vi "bresenham_algorithm.vi"(0 "pX":dbl, 5 "pY":dbl, 7 "speed (ms)":u32(knob) scale=0.0..20.0, 9 "newX":dbl, 11 "newY":dbl) -> ()   [LabVIEW 2016]
panel:
  out "error (dy > dx)":dbl
  out "error (dx >= dy)":dbl
  out "dX":dbl
  out "dY":dbl
  out "direction X":bool[](array[boolean])
  out "direction Y":bool[](array[boolean])
  # "This program let the user to draw a linear line at feed rate.\nThis program implement the Bresenham's line Algorithm. \nUser must enter feed rate in millisecond (ms).\nThe pX and pY is the start points of the linear line.\nThe newX and newY is the end points of the linear line."
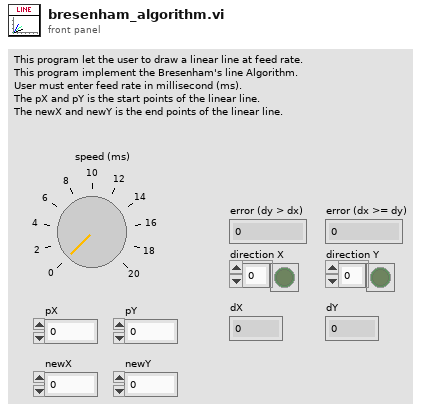
[diagram p1: front panel]
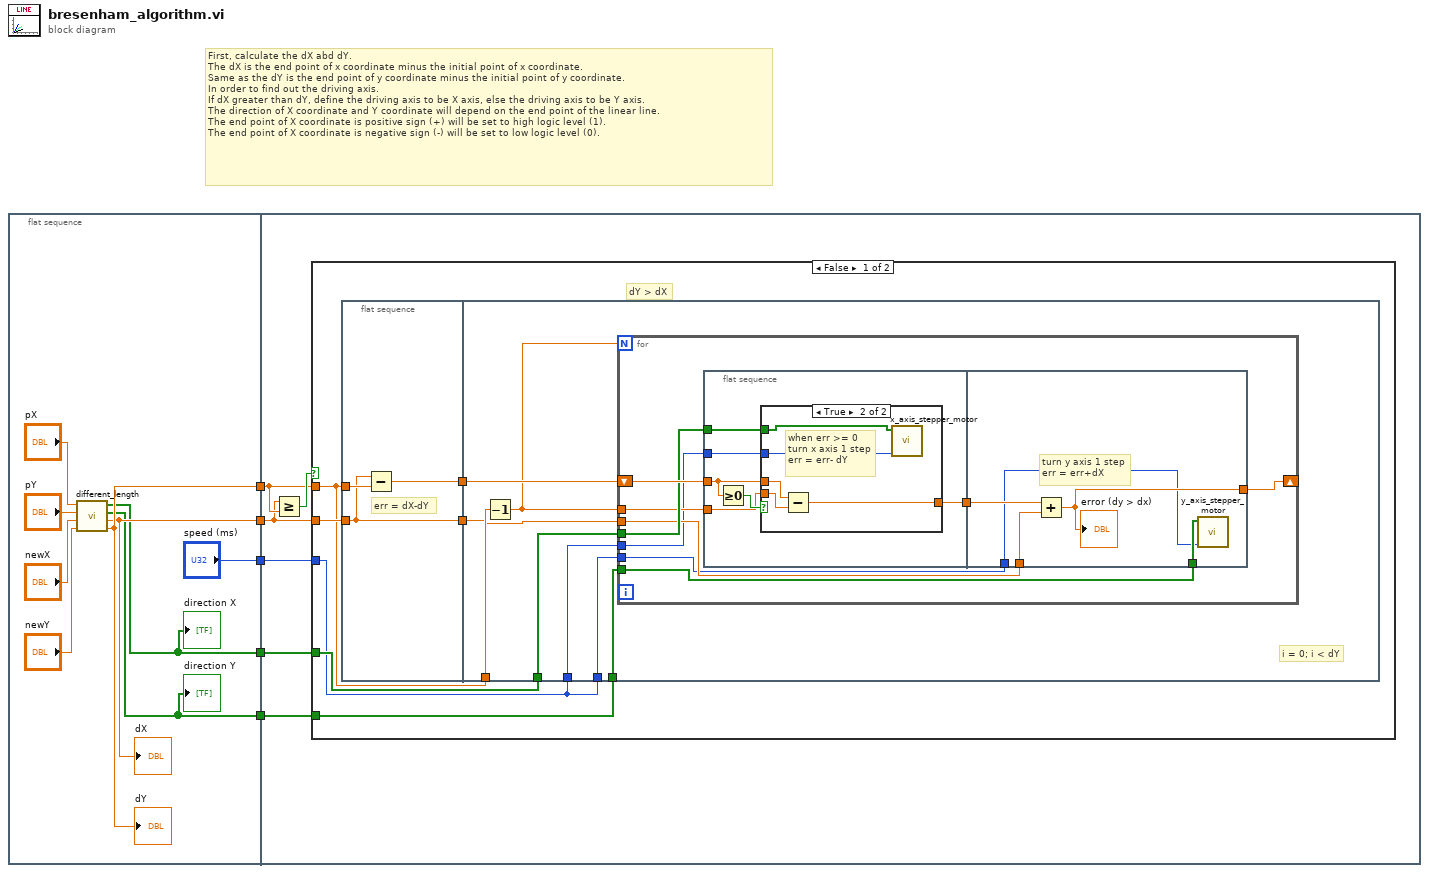
[diagram p0: block diagram]
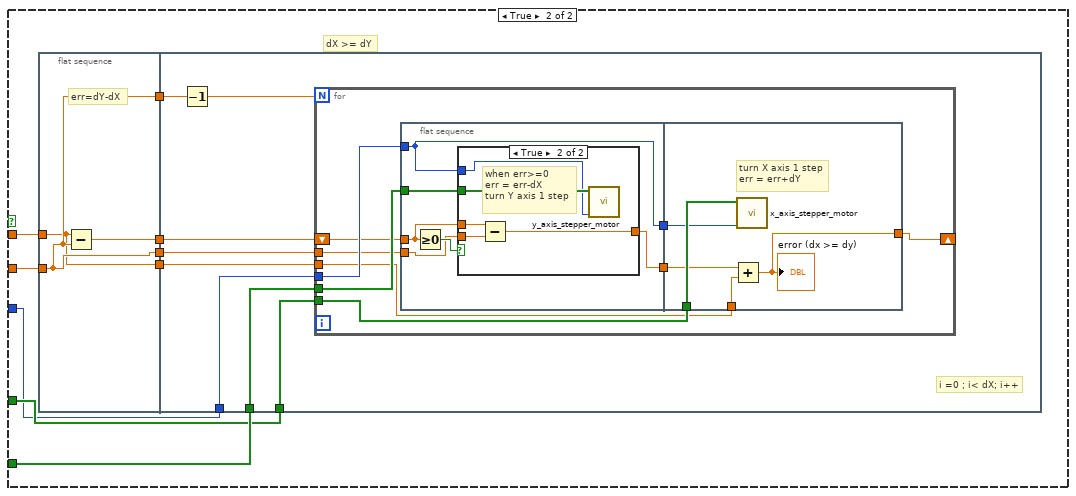
[diagram p3: hidden frame]
diagram:
  # "First, calculate the dX abd dY. \nThe dX is the end point of x coordinate minus the initial point of x coordinate.\nSame as the dY is the end point of y coordinate minus the initial point of y coordinate.\nIn order to find out the driving axis. \nIf dX greater than dY, define the driving axis to be X axis, else the driving axis to be Y axis.\nThe direction of X coordinate and Y coordinate will depend on the end point of the linear line. \nThe end point of X coordinate is positive sign (+) will be set to high logic level (1).\nThe end point of X coordinate is negative sign (-) will be set to low logic level (0)."
  n1 = flat-sequence {
    tunnel: [w12] -> w5
    tunnel: [w11] -> w4
    tunnel: [w10] -> w3
    tunnel: ["speed (ms)"] -> w2
    tunnel: [w13] -> w1
    tunnel: w5 -> [w15]
    tunnel: w4 -> [w19]
    tunnel: w3 -> [w18]
    tunnel: w2 -> [w17]
    tunnel: w1 -> [w16]
    frame #0 {
      n2 = call "different_length.vi"("newY"="newY", "newX"="newX", "pY"="pY", "pX"="pX") -> ("dY"=w13:dbl, "dX"=w12:dbl, "dirY"=w11:bool[], "dirX"=w10:bool[])  [unwired: 4 in]
      "dX" <- w12
      "dY" <- w13
      "direction X" <- w10
      "direction Y" <- w11
    }
    frame #1 {
      n3 = Greater Or Equal?(x=w15, y=w16) -> (x >= y?=w20:bool)
      n4 = case shown="False" w20 {
        tunnel: w19 -> [w26 w73]
        tunnel: w18 -> [w25 w72]
        tunnel: w17 -> [w21 w71]
        tunnel: w16 -> [w23 w69]
        tunnel: w15 -> [w24 w68]
        frame False {
          # "dY > dX"
          n5 = flat-sequence {
            tunnel: [w30] -> w27
            tunnel: w24 -> [w28]
            tunnel: w23 -> [w29]
            tunnel: [w28] -> w22
            tunnel: w27 -> [w38]
            tunnel: w26 -> [w37]
            tunnel: w25 -> [w36]
            tunnel: w23 -> [w35]
            tunnel: w22 -> [w33]
            tunnel: w21 -> [w32]
            tunnel: w21 -> [w31]
            frame #0 {
              # "err = dX-dY"
              n6 = Subtract(x=w28, y=w29) -> (x-y=w30:dbl)
            }
            frame #1 {
              # "i = 0; i < dY"
              n7 = Decrement(x=w35) -> (x-1=w34:dbl)
              n8 = for {
                N: w34 -> [_]
                shift-right: [w45] -> _
                shift-left: w38 -> [w47]
                tunnel: w36 -> [w44]
                tunnel: w37 -> [w43]
                tunnel: w34 -> [w42]
                tunnel: w33 -> [w41]
                tunnel: w32 -> [w40]
                tunnel: w31 -> [w39]
                n9 = flat-sequence {
                  tunnel: w47 -> [w52]
                  tunnel: [w51] -> w46
                  tunnel: w44 -> [w50]
                  tunnel: w42 -> [w49]
                  tunnel: w40 -> [w48]
                  tunnel: [w63] -> w45
                  tunnel: w46 -> [w64]
                  tunnel: w43 -> [w62]
                  tunnel: w41 -> [w61]
                  tunnel: w39 -> [w60]
                  frame #0 {
                    n10 = Greater Or Equal To 0?(x=w52) -> (x >= 0?=w53:bool)
                    n11 = case shown="True" w53 {
                      tunnel: w52 -> [w54 w59]
                      tunnel: [w54 w58] -> w51
                      tunnel: w50 -> [_ w57]
                      tunnel: w49 -> [_ w56]
                      tunnel: w48 -> [_ w55]
                      frame False {
                        # "do nothing"
                      }
                      frame True {
                        # "when err >= 0\nturn x axis 1 step\nerr = err- dY"
                        n12 = Subtract(x=w59, y=w56) -> (x-y=w58:dbl)
                        n13 = call "x_axis_stepper_motor.vi"("speed"=w55, "Direction"=w57) -> ()  [unwired: 10 in]
                      }
                    }
                  }
                  frame #1 {
                    # "turn y axis 1 step\nerr = err+dX"
                    n14 = Add(x=w64, y=w61) -> (x+y=w63:dbl)
                    "error (dy > dx)" <- w63
                    n15 = call "y_axis_stepper_motor.vi"("speed"=w60, "Direction"=w62) -> ()  [unwired: 10 in]
                  }
                }
              }
            }
          }
        }
        frame True {
          # "dX >= dY"
          n16 = flat-sequence {
            tunnel: [w76] -> w70
            tunnel: w69 -> [w74]
            tunnel: w68 -> [w75]
            tunnel: [w75] -> w67
            tunnel: [w75] -> w66
            tunnel: [w74] -> w65
            tunnel: w73 -> [w83]
            tunnel: w72 -> [w82]
            tunnel: w71 -> [w81]
            tunnel: w70 -> [w80]
            tunnel: w67 -> [w79]
            tunnel: w66 -> [w78]
            tunnel: w65 -> [w77]
            frame #0 {
              # "err=dY-dX"
              n17 = Subtract(x=w74, y=w75) -> (x-y=w76:dbl)
            }
            frame #1 {
              # "i =0 ; i< dX; i++"
              n18 = Decrement(x=w79) -> (x-1=w84:dbl)
              n19 = for {
                N: w84 -> [_]
                tunnel: w83 -> [w93]
                tunnel: w82 -> [w92]
                tunnel: w81 -> [w91]
                shift-right: [w87] -> _
                shift-left: w80 -> [w90]
                tunnel: w78 -> [w89]
                tunnel: w77 -> [w86]
                n20 = flat-sequence {
                  tunnel: w93 -> [w98]
                  tunnel: w91 -> [w94]
                  tunnel: w90 -> [w97]
                  tunnel: w89 -> [w96]
                  tunnel: [w95] -> w88
                  tunnel: [w94] -> w85
                  tunnel: w92 -> [w110]
                  tunnel: [w108] -> w87
                  tunnel: w88 -> [w109]
                  tunnel: w86 -> [w107]
                  tunnel: w85 -> [w106]
                  frame #0 {
                    n21 = Greater Or Equal To 0?(x=w97) -> (x >= 0?=w99:bool)
                    n22 = case shown="True" w99 {
                      tunnel: w98 -> [_ w105]
                      tunnel: w94 -> [_ w104]
                      tunnel: w97 -> [w100 w103]
                      tunnel: w96 -> [_ w102]
                      tunnel: [w100 w101] -> w95
                      frame False {
                        # "do nothing"
                      }
                      frame True {
                        # "when err>=0\nerr = err-dX\nturn Y axis 1 step"
                        n23 = Subtract(x=w103, y=w102) -> (x-y=w101:dbl)
                        n24 = call "y_axis_stepper_motor.vi"("speed"=w104, "Direction"=w105) -> ()  [unwired: 10 in]
                      }
                    }
                  }
                  frame #1 {
                    # "turn X axis 1 step\nerr = err+dY"
                    n25 = Add(x=w109, y=w107) -> (x+y=w108:dbl)
                    "error (dx >= dy)" <- w108
                    n26 = call "x_axis_stepper_motor.vi"("speed"=w106, "Direction"=w110) -> ()  [unwired: 10 in]
                  }
                }
              }
            }
          }
        }
      }
    }
  }
